vi "status of power_supply3.vi"() -> ()   [LabVIEW 2020]
panel:
  out "status of power_supply3":bool
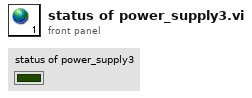
[diagram p1: front panel]
diagram:
